vi "readFromXML.vi"(8 "error in (no error)":errorcluster, 10 "XML in":string, 11 "OffsetCommands in":refnum<class "OffsetCommands.lvclass">) -> (0 "error out":errorcluster, 3 "OffsetCommands out":refnum<class "OffsetCommands.lvclass">)   [LabVIEW 2022 SP3, in "TCSDataDefinitions.lvlib" / "TCSCommand.lvlib" / "OffsetCommands.lvlib" / "OffsetCommands.lvclass"]
uses:
  OffsetCommands.lvclass
  TCSTcsCommand/TCSTcsCommand.lvclass
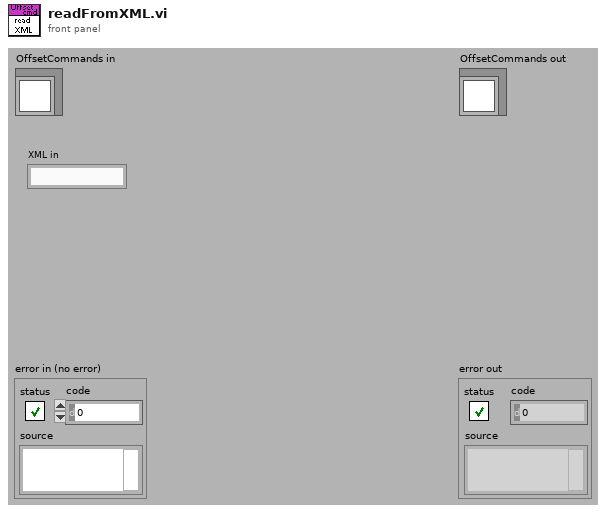
[diagram p1: front panel]
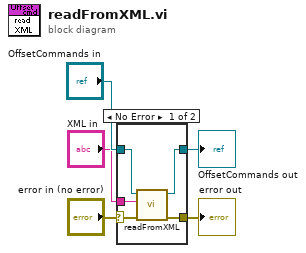
[diagram p0: block diagram]
diagram:
  n1 = case shown="No Error" "error in (no error)" {
    selector: "error in (no error)" -> [w8 w12]
    tunnel: [w7 w12] -> w4
    tunnel: [w6 w11] -> w2
    tunnel: "OffsetCommands in" -> [w9 w11]
    tunnel: "XML in" -> [w10 _]
    frame No Error {
      n2 = call-parent "readFromXML.vi"("error in (no error)"=w8, "XMLin"=w10, "TCSTcsCommand in"=w9) -> ("error out"=w7:errorcluster, "TCSTcsCommand out"=w6:refnum<class "OffsetCommands.lvclass">)  [unwired: 7 out]
    }
    frame Error {
    }
  }
  "error out" <- w4
  "OffsetCommands out" <- w2
